vi "Measure Diode Power.vi"(0 "COM Port in":refnum<visa-resource-name>, 1 "error in":errorcluster) -> (2 "COM Port out":refnum<visa-resource-name>, 3 "diode power":dbl, 4 "OK":bool, 5 "error out":errorcluster)   [LabVIEW 2013]
doc: "This command measures the actual laser power via the internal light pickoff.\nThis command is not valid for LEDMOD.v2 since it is not equipped with a light pickoff."
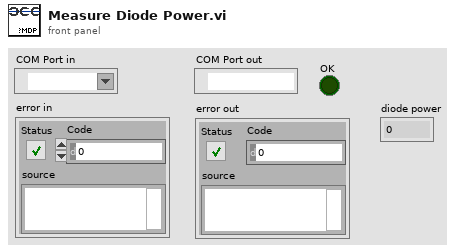
[diagram p1: front panel]
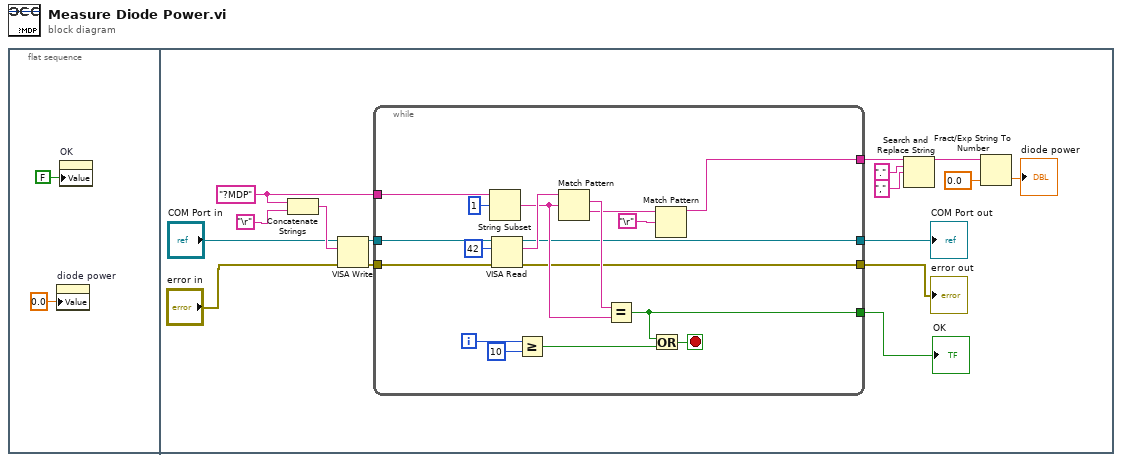
[diagram p0: block diagram]
diagram:
  n1 = flat-sequence {
    frame #0 {
      n2 = property on="diode power" class="DigWert (strikt)"("Value"=0.0 ("diode power")) -> ()  [unwired: 2 in, 2 out]
      n3 = property on="OK" class="Bool. (strikt)"("Value"=FALSE ("OK")) -> ()  [unwired: 2 in, 2 out]
    }
    frame #1 {
      w8 = "?MDP" ("Schreibpuffer")
      n4 = Concatenate Strings(w8, "\r") -> (w14:string)
      n5 = VISA Write(VISA resource name="COM Port in", write buffer=w14, error in (no error)="error in") -> (VISA resource name out=w12:refnum<visa-resource-name>, error out=w11:errorcluster)  [unwired: 1 out]
      n6 = while {
        tunnel: [w31] -> w18
        tunnel: [w30] -> w17
        tunnel: [w26] -> w7
        tunnel: w12 -> [w20]
        tunnel: w11 -> [w23]
        tunnel: w8 -> [w22]
        tunnel: [w21] -> w3
        i -> [w29]
        stop <- w24 stop-if-true
        n7 = String Subset(string=w22, offset (0)=1 ("Offset (0)")) -> (substring=w32:string)  [unwired: 1 in]
        n8 = VISA Read(VISA resource name=w20, byte count=u32 42 ("Byte-Anzahl"), error in (no error)=w23) -> (VISA resource name out=w31:refnum<visa-resource-name>, read buffer=w35:string, error out=w30:errorcluster)  [unwired: 1 out]
        n9 = Greater Or Equal?(x=w29, y=10) -> (x >= y?=w27:bool)
        n10 = Match Pattern(string=w35, regular expression=w32) -> (match substring=w34:string, after substring=w25:string)  [unwired: 1 in, 2 out]
        n11 = Equal?(x=w34, y=w32) -> (x = y?=w21:bool)
        n12 = Or(x=w21, y=w27) -> (x .or. y?=w24:bool)
        n13 = Match Pattern(string=w25, regular expression="\r") -> (before substring=w26:string)  [unwired: 1 in, 3 out]
      }
      "COM Port out" <- w18
      "error out" <- w17
      "OK" <- w3
      n14 = Search and Replace String(input string=w7, search string="." ("Such-String"), replace string="," ("String ersetzen(\"\")")) -> (result string=w6:string)  [unwired: 5 in, 3 out]
      n15 = Fract/Exp String To Number(string=w6, default (0 dbl)=0.0 ("Standard (0 I32)")) -> (number=→"diode power":dbl)  [unwired: 2 in, 1 out]
    }
  }
